vi "_Open Provider Reference.vi"(6 "password":string, 7 "type specifier VI Refnum":refnum<vi>, 8 "error in (no error)":errorcluster, 10 "vi path":path, 11 "application reference":refnum<vi>) -> (0 "error out":errorcluster, 3 "VI out":refnum<vi>)   [LabVIEW 2019, in "LabVIEW-ProviderShell.lvlib" / "LvProviderShellHelper.lvclass"]
uses:
  LvProviderShellHelper.lvclass
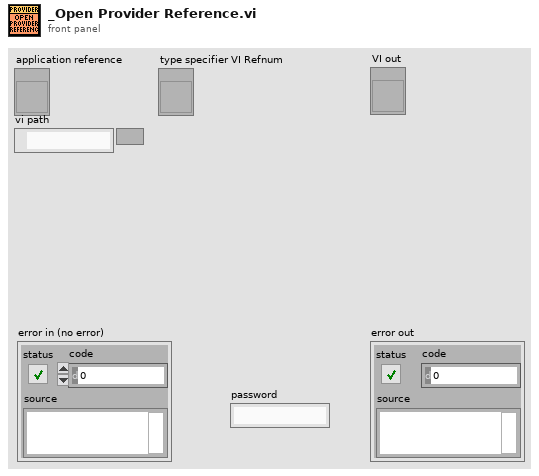
[diagram p1: front panel]
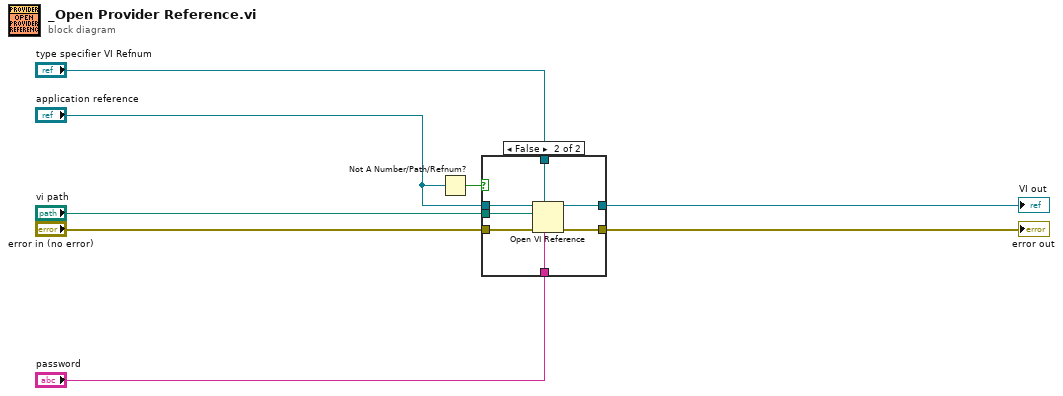
[diagram p0: block diagram]
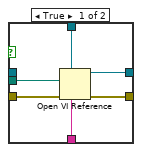
[diagram p2: hidden frame]
diagram:
  n1 = Not A Number/Path/Refnum?(number/path/refnum="application reference") -> (NaN/Path/Refnum?=w8:bool)
  n2 = case shown="False" w8 {
    tunnel: "vi path" -> [w14 w21]
    tunnel: [w13 w20] -> w2
    tunnel: [w12 w19] -> w3
    tunnel: "error in (no error)" -> [w11 w18]
    tunnel: "application reference" -> [_ w15]
    tunnel: "password" -> [w10 w17]
    tunnel: "type specifier VI Refnum" -> [w9 w16]
    frame True {
      n3 = Open VI Reference(type specifier VI Refnum (for type only)=w9, vi path=w14, password ("")=w10, error in (no error)=w11) -> (vi reference=w13:refnum<vi>, error out=w12:errorcluster)  [unwired: 2 in]
    }
    frame False {
      n4 = Open VI Reference(type specifier VI Refnum (for type only)=w16, application reference (local)=w15, vi path=w21, password ("")=w17, error in (no error)=w18) -> (vi reference=w20:refnum<vi>, error out=w19:errorcluster)  [unwired: 1 in]
    }
  }
  "error out" <- w3
  "VI out" <- w2
